vi "worksheet set comments author lv.vi"(8 "error in (no error)":errorcluster, 10 "author":string, 11 "worksheet":u32) -> (0 "error out":errorcluster)   [LabVIEW 2015, in "xlsxwriter.lvlib"]
doc: "void worksheet_set_comments_author_lv(lxw_worksheet worksheet, const char *author);"
uses:
  xlsxwriter.lvlib
  xlsxwriter.dll
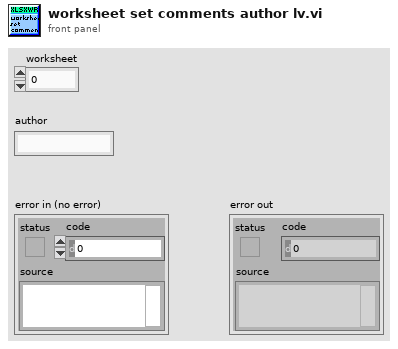
[diagram p1: front panel]
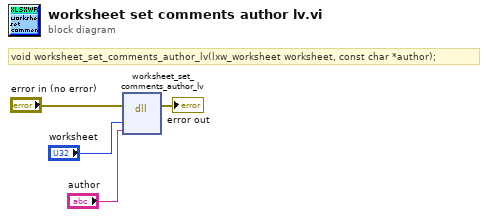
[diagram p0: block diagram]
diagram:
  # "void worksheet_set_comments_author_lv(lxw_worksheet worksheet, const char *author);"
  n1 = dll-call lib="C:/Users/WDAGUtilityAccount/Desktop/lv_vis_added_cell/xlsxwriter.*" fn="worksheet_set_comments_author_lv"(error in="error in (no error)", "worksheet"="worksheet", "author"="author") -> (error out=→"error out":errorcluster)  [unwired: 5 in, 1 out]
